vi "Vision Processing.vi"(4 "error in (no error)":errorcluster, 7 "Image Size":T4=enum."320x240") -> ()   [LabVIEW 2014]
doc: "This VI runs in parallel to other tasks. It gets images from the camera, processes them for color or shape and use that information to affect robot behavior."
uses:
  <vilib>/Rock Robotics/WPI/Camera/WPI_CameraImageSize.ctl
  <vilib>/Rock Robotics/WPI/Camera/WPI_CameraWhite Balance Values.ctl
  <vilib>/Rock Robotics/WPI/Camera/WPI_CameraExposure Values.ctl
  <vilib>/Rock Robotics/WPI/Camera/WPI_CameraFrameRate.ctl
  Robot Global Data.vi
panel:
  out "Found Totes":T1(array[cluster]) {"Normalized Rect"."Numeric 5" format="%#_2g"; "Normalized Rect"."Numeric 3" format="%#_2g"; "Normalized Rect"."Numeric 2" format="%#_2g"; "Normalized Rect"."Numeric" format="%#_2g"}
  out "Sorted Scores":T2(array[cluster]) {"Correlation" format="%#_3g"; "Scale %" format="%#_3g"; "Score" format="%#_3g"}
  out "Particles":i32
  in  "Tote Color":T3={"Hue"={23.67058792990901, 48.923317529462665}, "Sat"={66.78571428571429, 255.0}, "Val"={48.571428571428584, 255.0}} {"Hue" scale=0.0..255.0 scale format="%#_3g"}
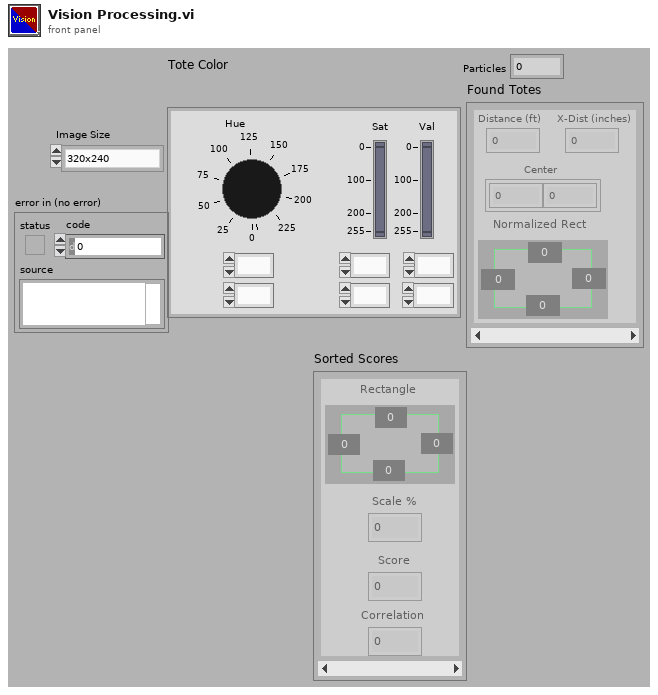
[diagram p1: front panel]
types:
  T1 = cluster{"Distance (ft)":dbl, "X-Dist (inches)":dbl, "Center":cluster{dbl, dbl}, "Normalized Rect":cluster{"Numeric":dbl, "Numeric 2":dbl, "Numeric 3":dbl, "Numeric 5":dbl}}[]
  T2 = cluster{"Rectangle":cluster{"Numeric":dbl, "Numeric 2":dbl, "Numeric 3":dbl, "Numeric 5":dbl}, "Scale %":dbl, "Score":dbl, "Correlation":dbl}[]
  T3 = cluster{"Hue":cluster{dbl, dbl}, "Sat":cluster{dbl, dbl}, "Val":cluster{dbl, dbl}}
  T4 = typedef "WPI_CameraImageSize.ctl" = enum16{"640x480", "320x240", "160x120", "Custom"}
  T5 = typedef "WPI_CameraFrameRate.ctl" = u32
  T6 = typedef "WPI_CameraExposure Values.ctl" = enum16{"Auto", "Flicker-free 50 Hz", "Flicker-free 60 Hz", "Hold current", "Custom"}
  T7 = typedef "WPI_CameraWhite Balance Values.ctl" = enum16{"Auto", "Fixed indoor", "Fixed outdoor 1", "Fixed outdoor 2", "Fixed fluorescent 1", "Fixed fluorescent 2", "Hold current", "Custom"}
  T8 = typedef "Image Type" = u32
  T9 = typedef "WPI_CameraDevRef.ctl" = cluster{"Camera Address":string, "CameraStatus":errorcluster}
  T10 = typedef "IMAQ Image.ctl" = refnum<image>
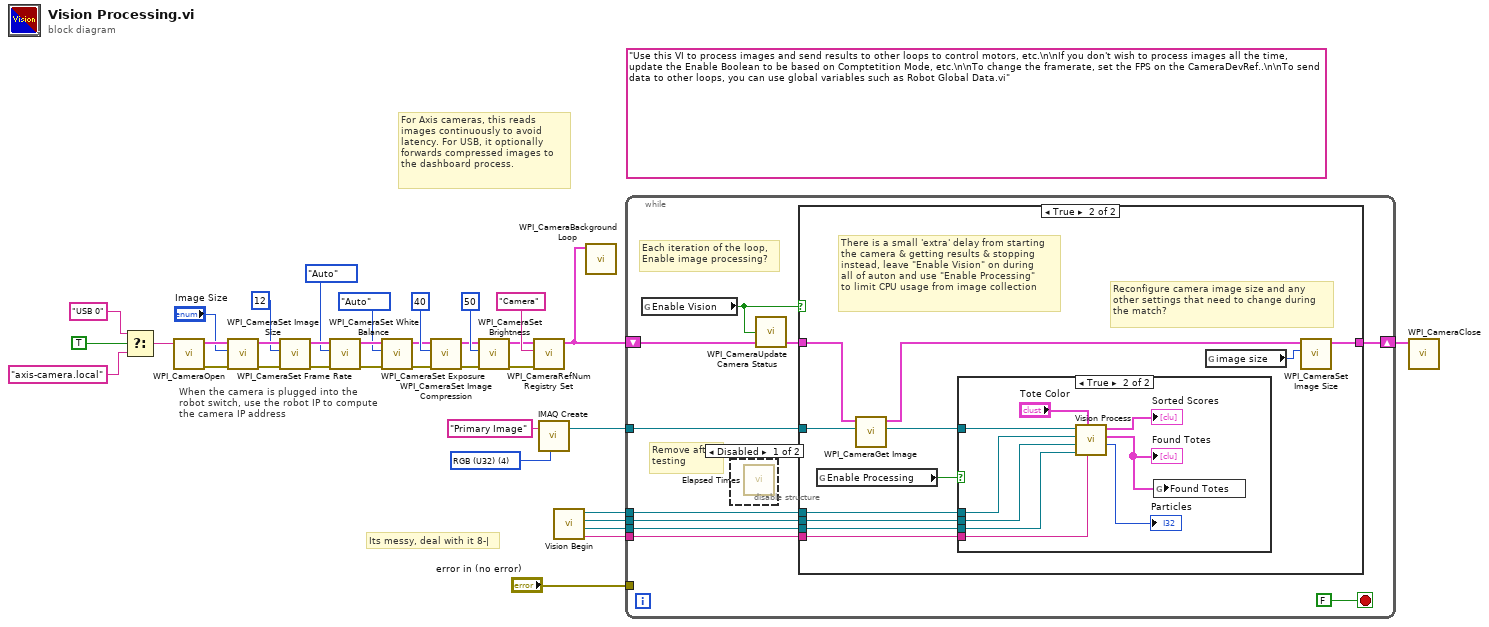
[diagram p0: block diagram]
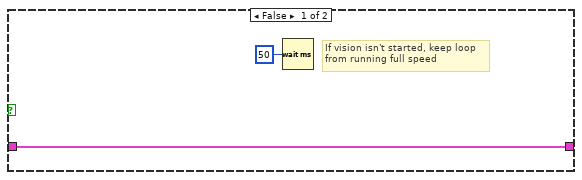
[diagram p3: hidden frame]
diagram:
  (unwired) "Use this VI to process images and send results to other loops to control motors, etc.\n\nIf you don't wish to process images all the time, update the Enable Boolean to be based on Comptetition Mode, etc.\n\nTo change the framerate, set the FPS on the CameraDevRef..\n\nTo send data to other loops, you can use global variables such as Robot Global Data.vi"
  w35 = T8 4 items=["Grayscale (U8)", "Grayscale (I16)", "Grayscale (SGL)", "Complex (CSG)", "RGB (U32)", "HSL (U32)", "RGB (U64)"] ("Image Type")
  # "Its messy, deal with it 8-|"
  # "When the camera is plugged into the\nrobot switch, use the robot IP to compute\nthe camera IP address"
  # "For Axis cameras, this reads\nimages continuously to avoid\nlatency. For USB, it optionally\nforwards compressed images to\nthe dashboard process."
  n1 = Select(t="USB 0" ("format string"), s=TRUE ("dot notation? (F)"), f="axis-camera.local" ("format string")) -> (s? t:f=w6:string)
  n2 = call <vilib>:"WPI_CameraOpen.vi"("Camera Address"=w6) -> ("error out"=w23:errorcluster, "CameraDevRef"=w24:T9)  [unwired: 1 in, 8 out]
  n3 = call <vilib>:"WPI_CameraSet Image Size.vi"("error in (no error)"=w23, "Image Size"="Image Size", "CameraDevRef"=w24) -> ("error out"=w22:errorcluster, "CameraDevRef Out"=w25:T9)  [unwired: 1 in, 6 out]
  n4 = call <vilib>:"WPI_CameraSet Frame Rate.vi"("error in (no error)"=w22, "Frame Rate (fps)"=T5 12, "CameraDevRef"=w25) -> ("error out"=w21:errorcluster, "CameraDevRef Out"=w27:T9)  [unwired: 7 out]
  n5 = call <vilib>:"WPI_CameraSet White Balance.vi"("error in (no error)"=w21, "White Balance"=WPI_CameraWhite_Balance_Values."Auto", "CameraDevRef"=w27) -> ("error out"=w20:errorcluster, "CameraDevRef Out"=w26:T9)  [unwired: 1 in, 6 out]
  n6 = call <vilib>:"WPI_CameraSet Exposure.vi"("error in (no error)"=w20, "Exposure"=WPI_CameraExposure_Values."Auto", "CameraDevRef"=w26) -> ("error out"=w19:errorcluster, "CameraDevRef Out"=w29:T9)  [unwired: 1 in, 6 out]
  n7 = call <vilib>:"WPI_CameraSet Image Compression.vi"("error in (no error)"=w19, "Compression"=40, "CameraDevRef"=w29) -> ("error out"=w18:errorcluster, "CameraDevRef Out"=w28:T9)  [unwired: 7 out]
  n8 = call <vilib>:"WPI_CameraSet Brightness.vi"("error in (no error)"=w18, "Brightness"=50, "CameraDevRef"=w28) -> ("error out"=w16:errorcluster, "CameraDevRef Out"=w17:T9)  [unwired: 7 out]
  n9 = call <vilib>:"WPI_CameraRefNum Registry Set.vi"("error in (no error)"=w16, "refnum name"="Camera", "CameraDevRef"=w17) -> ("CameraDevRef"=w12:T9)  [unwired: 8 out]
  n10 = call "IMAQ Create"("Image Name"="Primary Image", "Image Type"=w35) -> ("New Image"=w33:T10)  [unwired: 2 in, 2 out]
  n11 = call "Vision Begin.vi"() -> ("Match Geometric Pattern 2 Setup Data"=w2:string, "Gray Image"=w3:T10, "Tempalte"=w4:T10, "Mask"=w1:T10)  [unwired: 8 in]
  n12 = call <vilib>:"WPI_CameraBackground Loop.vi"("CameraDevRef"=w12) -> ()  [unwired: 11 in]
  n13 = while {
    shift-right: [w44] -> w10
    shift-left: w12 -> [w42]
    tunnel: w33 -> [w43]
    tunnel: "error in (no error)" -> [_]
    tunnel: w4 -> [w40]
    tunnel: w3 -> [w39]
    tunnel: w2 -> [w38]
    tunnel: w1 -> [w37]
    stop <- FALSE stop-if-true
    # "Remove after\ntesting"
    # "Each iteration of the loop,\nEnable image processing?"
    n14 = global read "Robot Global Data.vi" "Enable Vision"() -> (w36:bool)
    n15 = disable-structure shown="Disabled" {
      frame Disabled {
        n16 = call "Elapsed Times.vi"() -> ()  [unwired: 3 in, 1 out]
      }
      frame Enabled {
      }
    }
    n17 = call <vilib>:"WPI_CameraUpdate Camera Status.vi"("CameraDevRef In"=w42, "Enable Vision"=w36) -> ("CameraDevRef Out"=w41:T9)  [unwired: 3 in]
    n18 = case shown="True" w36 {
      tunnel: w43 -> [_ w57]
      tunnel: [w47 w58] -> w44
      tunnel: w41 -> [w47 w55]
      tunnel: w40 -> [_ w51]
      tunnel: w39 -> [_ w50]
      tunnel: w38 -> [_ w49]
      tunnel: w37 -> [_ w52]
      frame False {
        # "If vision isn't started, keep loop\nfrom running full speed"
        n19 = Wait (ms)(milliseconds to wait=u32 50) -> ()  [unwired: 1 out]
      }
      frame True {
        # "There is a small 'extra' delay from starting\nthe camera & getting results & stopping\ninstead, leave \"Enable Vision\" on during\nall of auton and use \"Enable Processing\"\nto limit CPU usage from image collection"
        # "Reconfigure camera image size and any\nother settings that need to change during\nthe match?"
        n20 = global read "Robot Global Data.vi" "Enable Processing"() -> (w48:bool)
        n21 = call <vilib>:"WPI_CameraGet Image.vi"("Image"=w57, "CameraDevRef"=w55) -> ("Image Out"=w53:T10, "CameraDevRef Out"=w54:T9)  [unwired: 1 in, 7 out]
        n22 = case shown="True" w48 {
          tunnel: w53 -> [_ w67]
          tunnel: w52 -> [_ w66]
          tunnel: w51 -> [_ w65]
          tunnel: w50 -> [_ w64]
          tunnel: w49 -> [_ w63]
          frame False {
          }
          frame True {
            n23 = call "Vision Process.vi"("Match Geometric Pattern 2 Setup Data"=w63, "Tote Color"="Tote Color", "Gray"=w64, "Template"=w65, "Mask"=w66, "Camera In"=w67) -> ("Particles"=→"Particles":i32, "Found Totes"=w59:T1, "Sorted Scores"=→"Sorted Scores":T2)  [unwired: 3 in]
            "Found Totes" <- w59
            n24 = global write "Robot Global Data.vi" "Found Totes"(w59) -> ()
          }
        }
        n25 = global read "Robot Global Data.vi" "image size"() -> (w56:T4)
        n26 = call <vilib>:"WPI_CameraSet Image Size.vi"("Image Size"=w56, "CameraDevRef"=w54) -> ("CameraDevRef Out"=w58:T9)  [unwired: 2 in, 7 out]
      }
    }
  }
  n27 = call <vilib>:"WPI_CameraClose.vi"("CameraDevRef"=w10) -> ()  [unwired: 1 in, 10 out]
